vi "判定大小数.vi"() -> ()   [LabVIEW 2015]
panel:
  in  "stop":bool
  out "循环次数":dbl
  out "小数":dbl
  out "大数":dbl
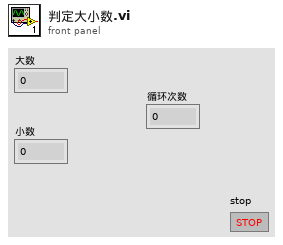
[diagram p1: front panel]
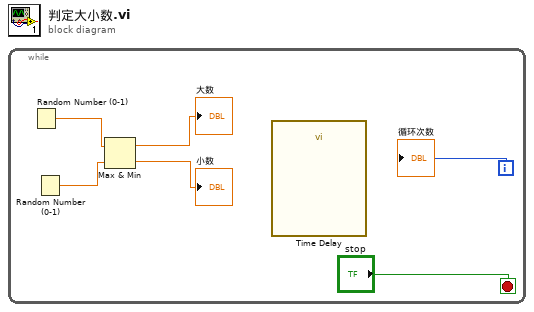
[diagram p0: block diagram]
diagram:
  n1 = while {
    i -> [w2]
    stop <- "stop" stop-if-true
    n2 = Random Number (0-1)() -> (number: 0 to 1=w6:dbl)
    n3 = Random Number (0-1)() -> (number: 0 to 1=w5:dbl)
    n4 = Max & Min(x=w6, y=w5) -> (max(x,y)=→"大数":dbl, min(x,y)=→"小数":dbl)
    n5 = call "Time Delay"() -> ()  [unwired: 11 in, 1 out]
    "循环次数" <- w2
  }
